vi "CCD_config.vi"() -> ()   [LabVIEW 2014]
uses:
  Public/Documents/SIToolkit/LabVIEW/Examples2014_6_0_2_9/Fast Examples/Open-Close Hardware/CamHandle.vi
  <vilib>/Utility/file.llb/Write To Spreadsheet File (I64).vi
  <vilib>/Utility/file.llb/Write To Spreadsheet File (DBL).vi
panel:
  in  "?":enum32{"CONFIGERATION", "OPERATION"}(tab)
  in  "Bypass Cooling":bool
  out "Camera Open":bool=TRUE
  in  "Write Tab Control":T1(tab)=enum."ROI"
  in  "Frames to collect (nframe)":u32=1 min=1 step=1
  in  "Exposure":dbl min=0.0 step=0.001 format="%.3f"
  in  "Timing Mode":u32(ring)=3 items=["Free Run/Timed"=1, "External Sync"=3, "Shift per Trigger"=13]
  in  "Trigger Edge":u32(ring)=1 items=["Positive Edge"=1, "Negative Edge"=2]
  in  "Collection Mode":u32(ring)=1 items=["Focus"=1, "N-Frame"=2, "Asynchronous"=3]
  in  "ReadOut Mode":u16(ring)=1 items=["Full Frame"=1, "Kinetics"=10]
  in  "Temperature":dbl=-75.0 format="%.2f"
  in  "Speed":i32=-2 min=-3 step=1
  in  "Gain":i32(ring)=1 items=["Don't Change "=-1, "Low"=1, "Medium"=2, "High"=3]
  in  "Offset":i32=-1 min=-1 step=1
  in  "Readout Port":i32(ring)=2 items=["Don't Change"=-1, "Low Noise"=1, "High capacity"=2]
  in  "Open":u32
  in  "Close":u32
  in  "Shutter State":u16(ring)=3 items=["Always Closed"=1, "Open Each Exposure"=2, "Open at Begining of Acquisition"=3, "Open While Waiting for Trigger"=4]
  in  "Final Section Height\n(Minimum Block Size)":u32=100
  in  "Final Section Count\n(Number of Minimum Blocks)":u32=10
  in  "Number of Clean/Clears cycles":u32
  in  "Clean cycle height (Number of \nStrips per Clean/Clear)":u32=100
  in  "Continous Cleans":bool
  in  "Skip Serial Register Clean":bool
  in  "Kinetics Window Height":u32
  in  "Active Y Size":u32=100
  in  "Post Y":u32=8
  in  "Pre Y":u32=8
  in  "Active X Size":u32=1340
  in  "Post X":u32
  in  "Pre X":u32
  in  "Vertical Timing Index":u32
  in  "Enable / Disable Custom Chip":bool
  in  "Logic Output":u16(ring)=3 items=["Not Scan / Not Reading"=1, "Shutter Open"=2, "Not Ready/Busy"=3, "Always Low"=4, "Always High"=8]
  in  "Invert":bool
  out "Y Size ROI":u32=100
  out "X Size ROI":u32=1340
  in  "Y Bin":u32=100 min=1 step=1
  in  "Y End":u32=100 min=1 step=1
  in  "Y Start":u32=1 min=1 step=1
  in  "X Bin":u32=1 min=1 step=1
  in  "X End":u32=1340 min=1 max=100000 step=1
  in  "X Start":u32=1 min=1 step=1
  in  "Camera Number":u32=1
  in  "Error Codes":string="Ready"
  out "Frame Rate Calc":dbl=1001.0010010010011
  out "Vertical Index":u32
  out "Custom Chip Enabled":bool
  out "Vertical Timing":dbl=3.2
  out "Readout Time":dbl=0.9989999999999999
  out "Temperature":dbl=-66.0
  out "Pixel Time\n(1/ADC Speed)":i32=500
  out "Bit Depth":i32=16
  out "ReadOut Port":i32=2
  out "ADC Offset":i32=-1
  out "ADC Gain":i32=1
  out "ADC Speed":i32=2000
  in  "error in (no error)":errorcluster
  out "error out":errorcluster
  out "Camera Handle":u32
  in  "INI Flag":bool=TRUE
  in  "Run":enum32{"RUN", "FOCUS", "FSRS", "SPECTROGRAPH"}(tab)
  in  "?":bool
  in  "Exposure Time (s)":dbl=0.004 min=0.0 step=0.001 format="%.3f"
  in  "?":bool
  in  "?":bool
  out "?":u16[](graph)
  in  "file path":path
  in  "File_name":string
  in  "# of spectrum per frame":i32
  in  "# of Frames":i32
  out "Gain":dbl
  in  "FLIP SPECTRA":bool
  in  "?":bool
  in  "?":bool
  in  "?":bool
  out "Spectra":dbl[](graph)
  in  "?":bool
  in  "Number of Images":u32=1 min=1 step=1
  out "DATA LOOP":dbl
  out "?":dbl[](graph)
  in  "?":bool
  in  "# of Sets":i32
  out "Current Set":u32=24
  in  "#Ground per set":u32=3
  in  "Timepoints":dbl[](array[numeric])=[200.0, 100.0, 300.0, 400.0, 500.0]
  in  "File Path":path
  in  "File Name":string
  in  "Ground State\nSubstract?":bool
  in  "?":bool
  out "Ready to Run":bool
  # "Timing"
  # "Seconds"
  # "Temperature"
  # "°C"
  # "ADC"
  # "-3 = SLOWEST speed\n-2 = FASTEST speed\n-1 = CURRENT speed (or do not wire)\nOtherwise enter speed in kHz"
  # "Shutter"
  # "Compensation Times"
  # "ms"
  # "Cleans / Clears"
  # "Custom Chip and Timing"
  # "Valid When Kinetics Timing Mode Active"
  # "Logic Output"
  # "Region Of Interest"
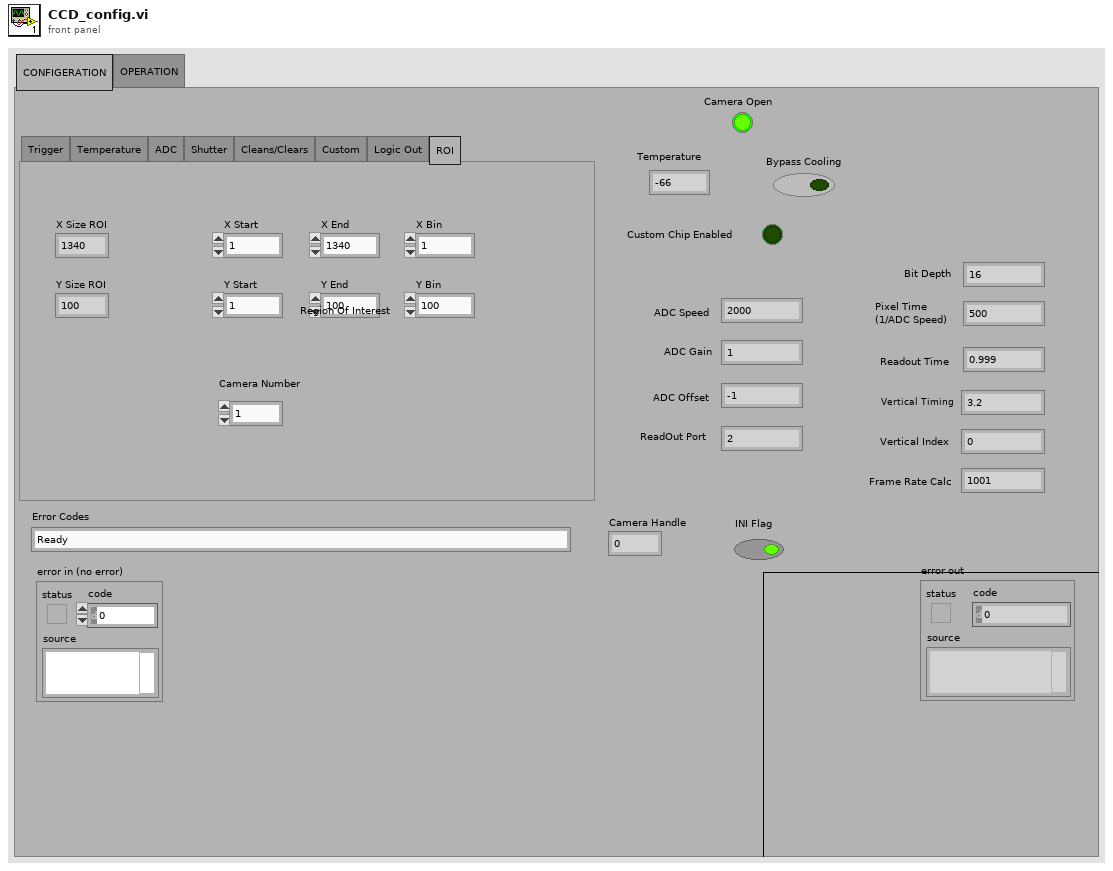
[diagram p1: front panel]
types:
  T1 = enum32{"Trigger", "Temperature", "ADC", "Shutter", "Cleans/Clears", "Custom", "Logic Out", "ROI"}
  T2 = enum8{"Enabled", "Disabled", "Disabled and Grayed Out"}
  T3 = cluster{"Camera Number":i32, "ROI Number":i32, "X Start":i32, "X End":i32, "X Bin":i32, "Y Start":i32, "Y End":i32, "Y Bin":i32}
  T4 = cluster{"Pre Y":u32, "Post Y":u32, "Active Y":u32, "Pre X":u32, "Post X":u32, "Active X":u32, "Custom Chip Enabled":bool, "Vertical Timing Index":u32}
  T5 = cluster{"Exposure":dbl, "Collection Mode":u32, "Timing Mode":u32, "Trigger Edge":u32, "Temperature":dbl}
  T6 = cluster{"ADC Speed":i32, "ADC Gain":i32, "ADC Offset":i32, "Readout Port":i32, "Num Cleans":u32, "Num Strips per Clean":u32, "Mini Block Size":u32, "Num Min Blocks":u32, "Continous Cleans":bool, "Skip Serial Reg Clean":bool}
  T7 = cluster{"Shutter State":u16, "Open Comp Time ":u32, "Close Comp Time":u32, "Logic Out Setting":u32, "Logic Out Invert":bool}
  T8 = cluster{"acquire focus mode":u32, "Exposure Time (s)":dbl, i32, "Software accumulation":u32}
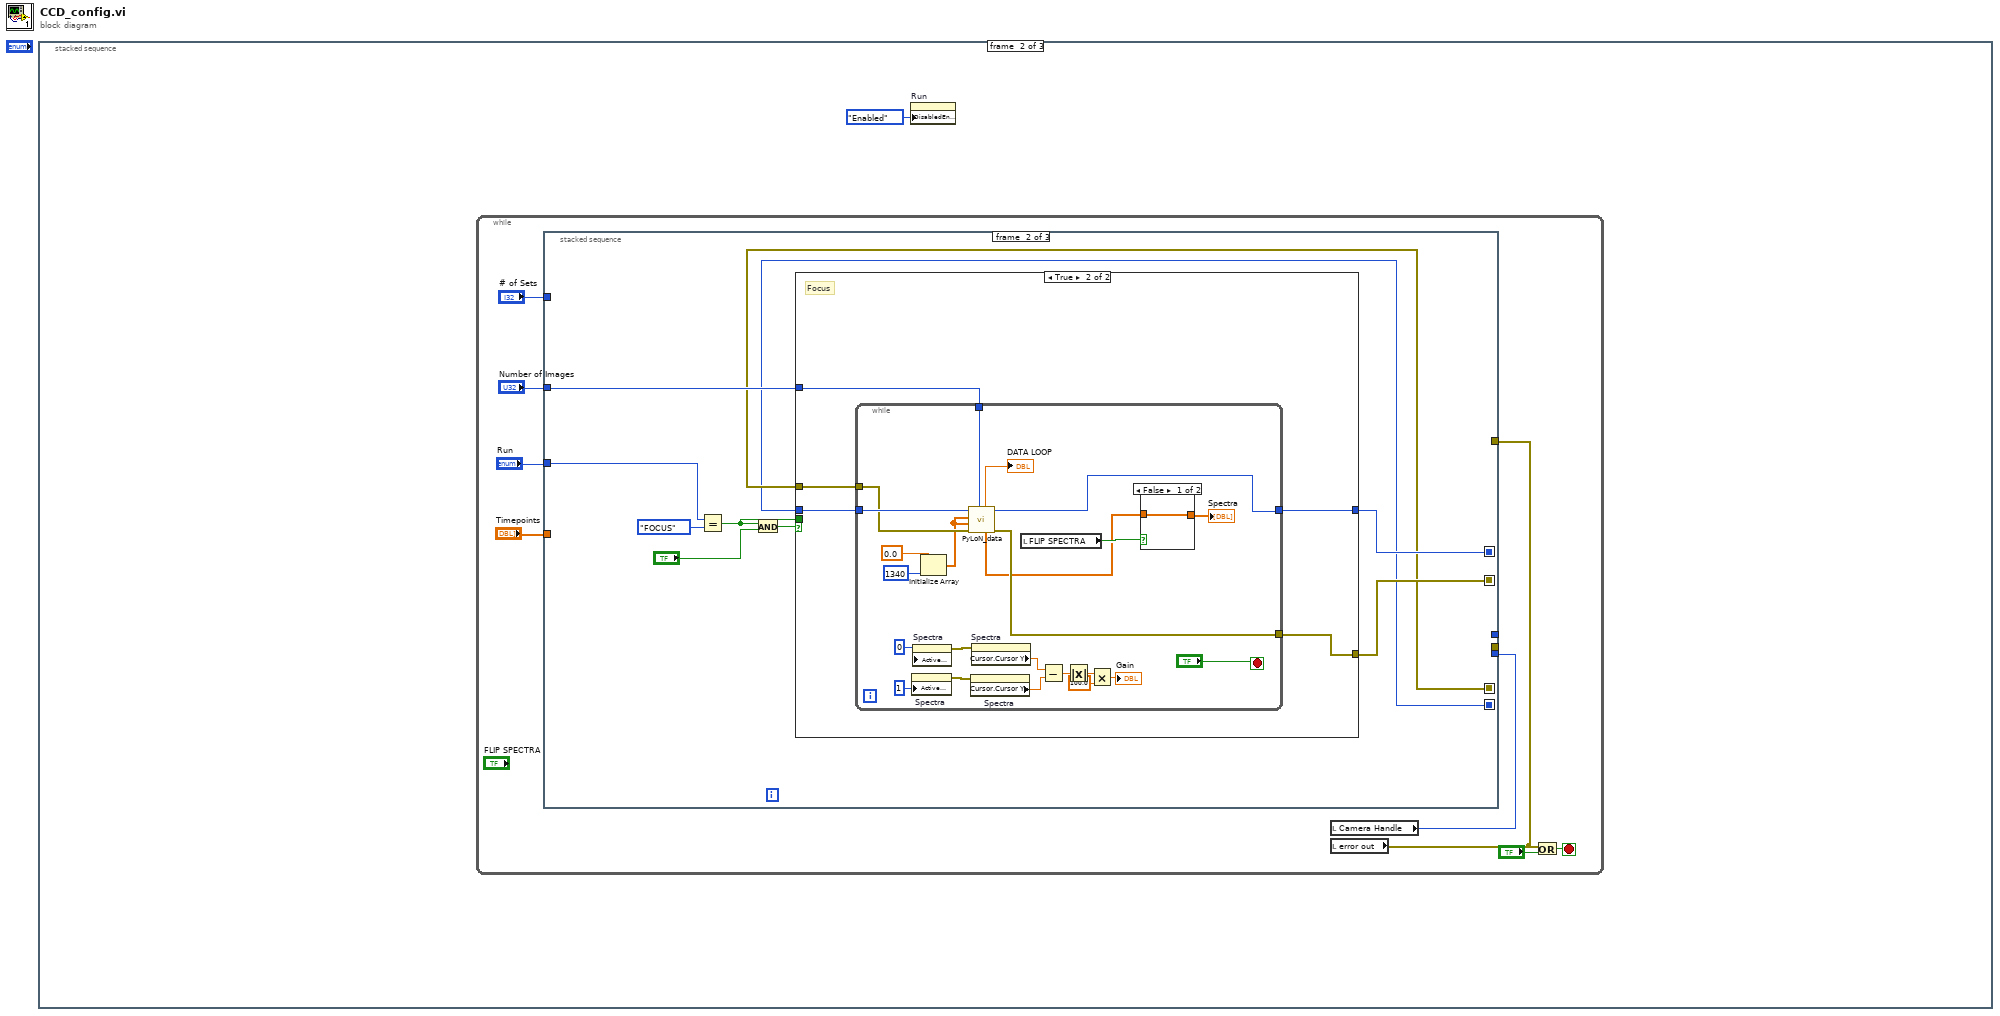
[diagram p0: block diagram]
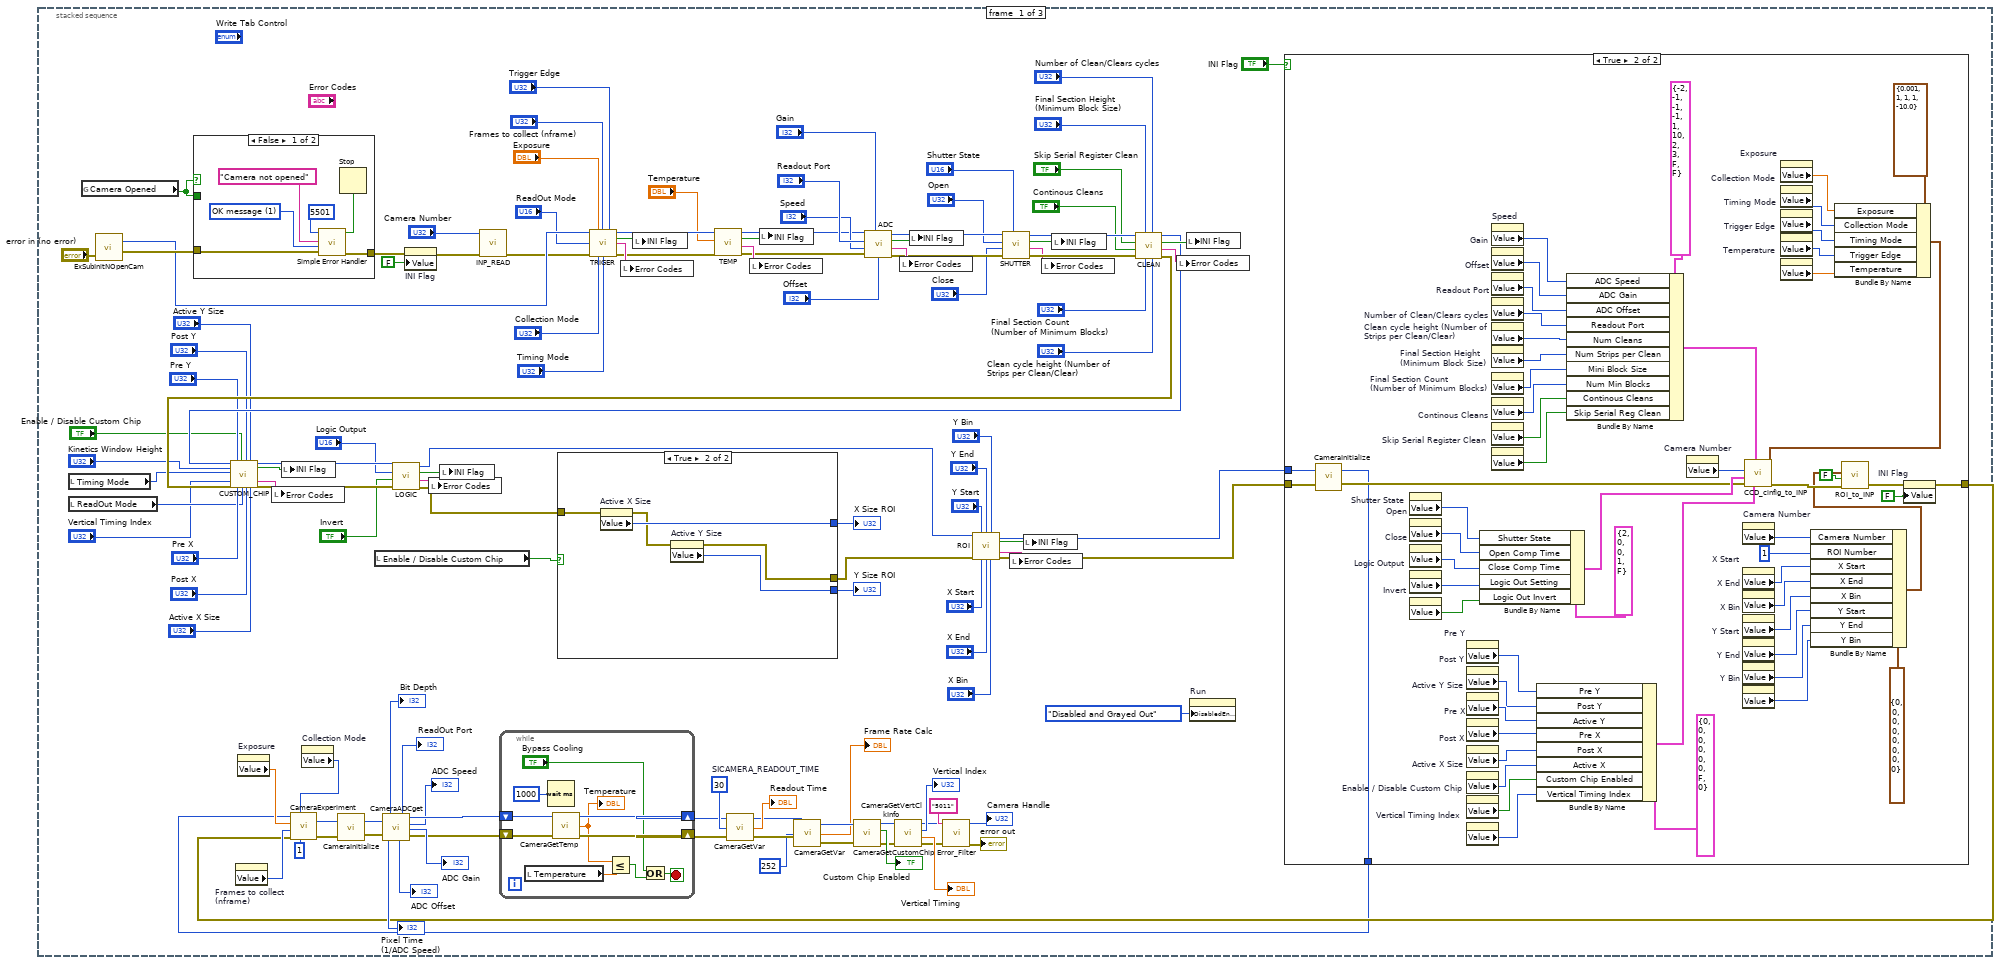
[diagram p2: hidden frame]
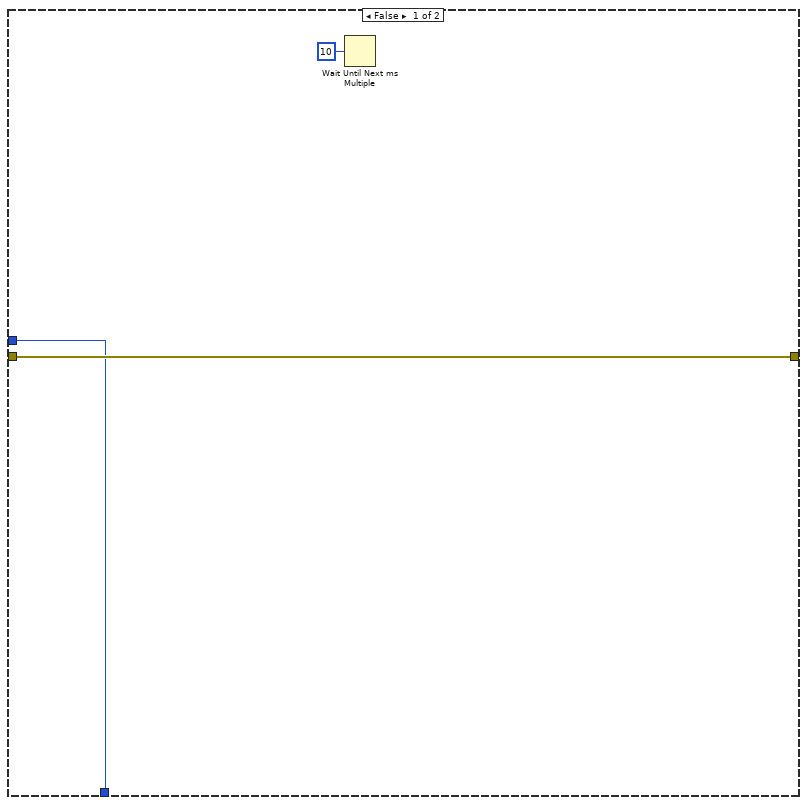
[diagram p3: hidden frame]
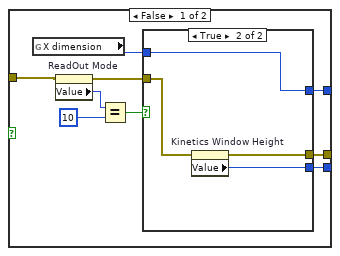
[diagram p4: hidden frame]
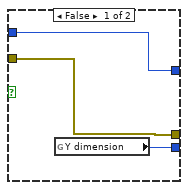
[diagram p5: hidden frame]
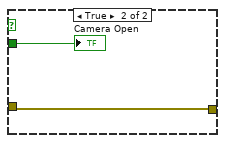
[diagram p6: hidden frame]
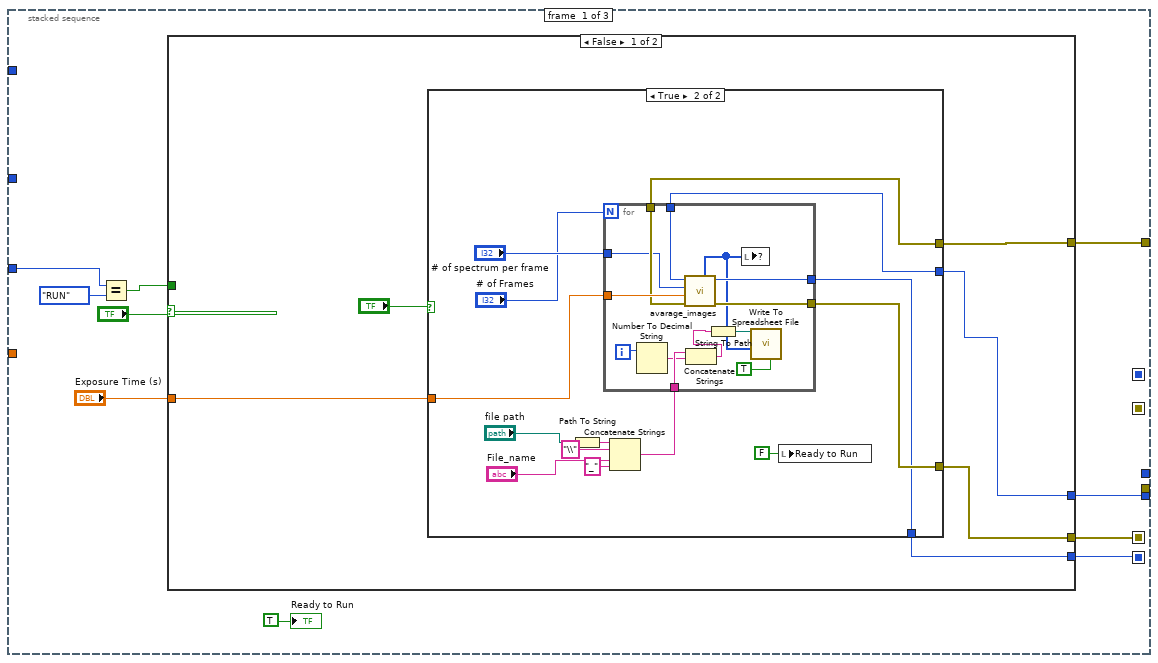
[diagram p7: hidden frame]
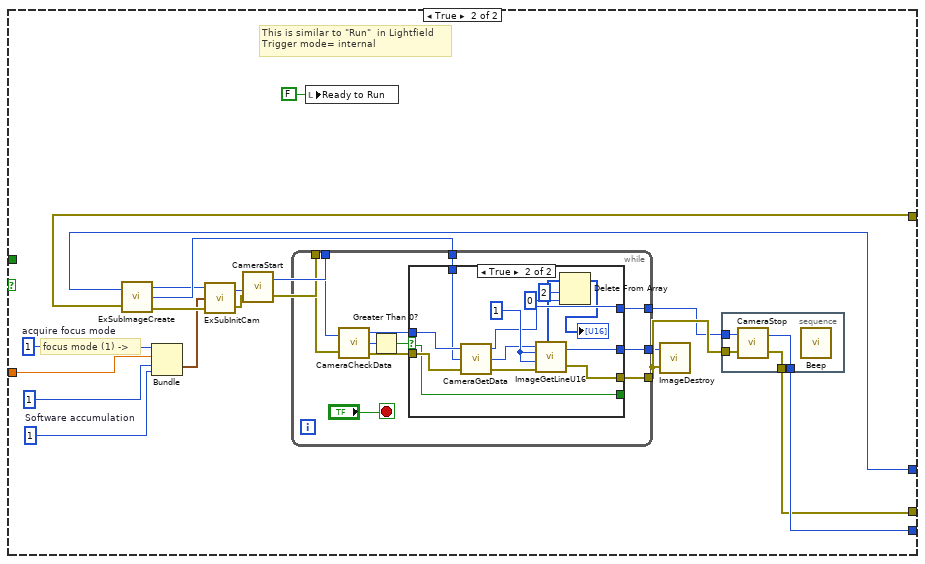
[diagram p9: hidden frame]
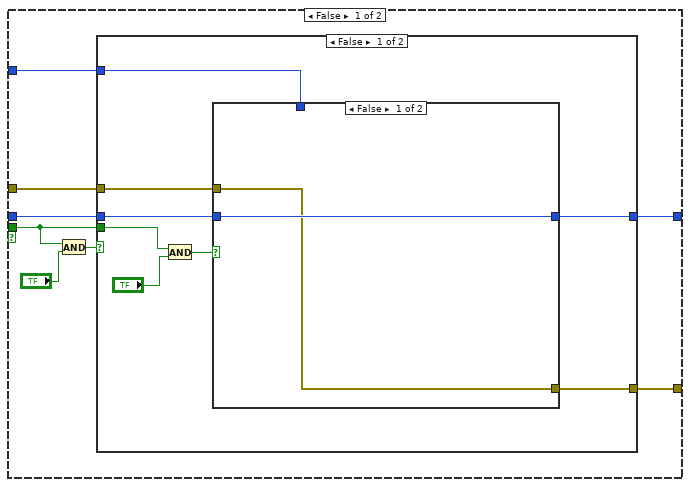
[diagram p11: hidden frame]
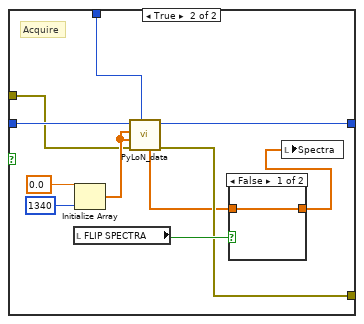
[diagram p12: hidden frame]
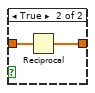
[diagram p13: hidden frame]
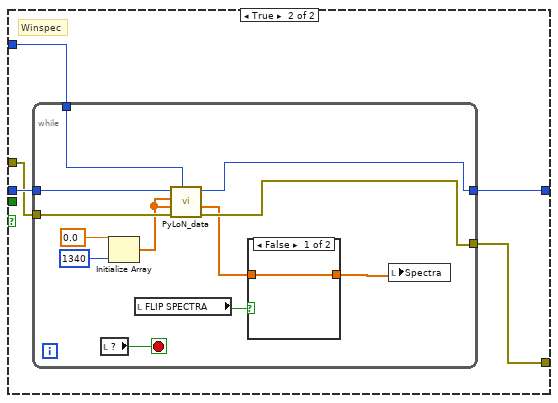
[diagram p14: hidden frame]
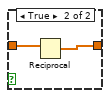
[diagram p15: hidden frame]
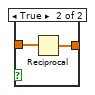
[diagram p16: hidden frame]
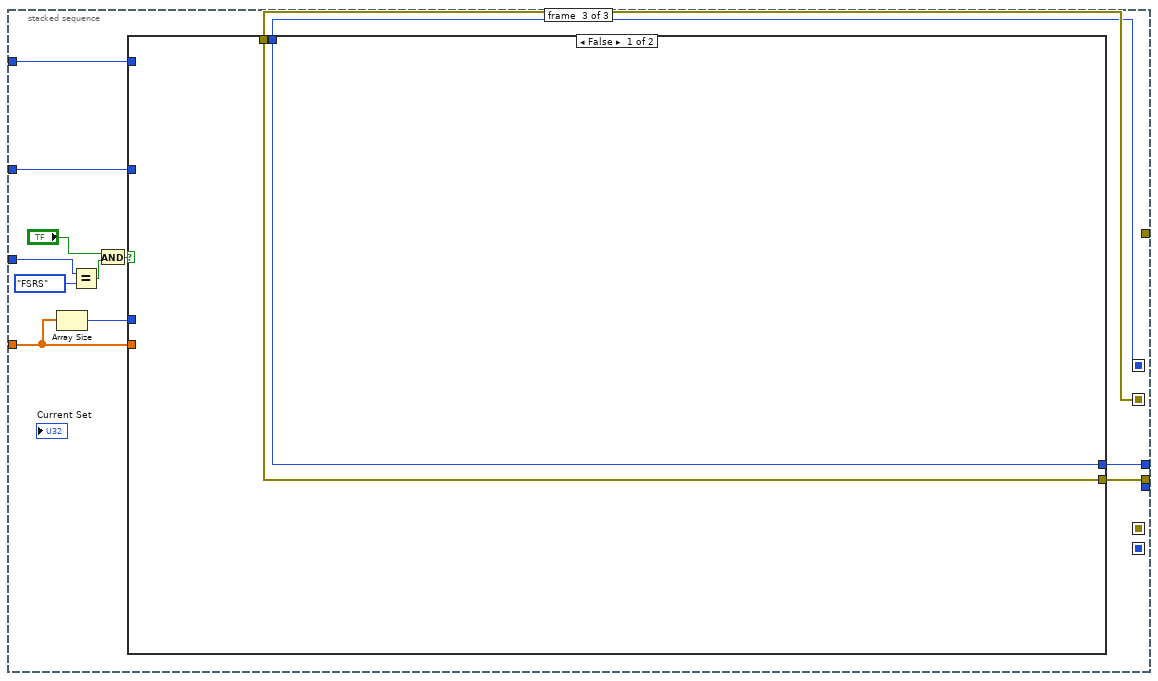
[diagram p17: hidden frame]
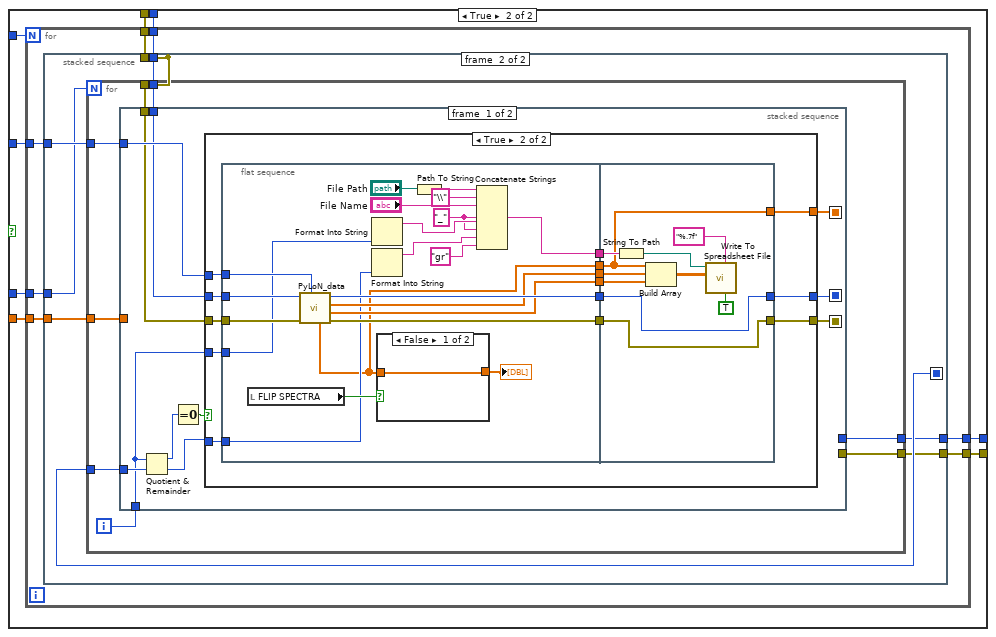
[diagram p18: hidden frame]
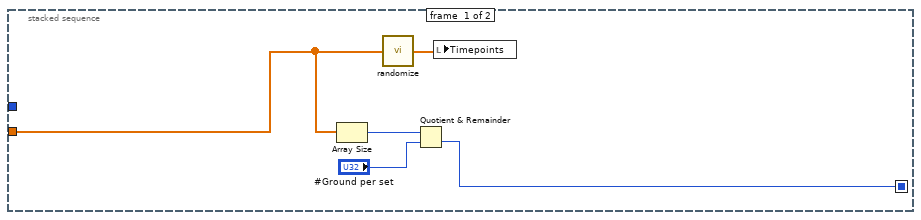
[diagram p19: hidden frame]
diagram:
  n1 = stacked-sequence {
    frame #0 {
      w33 = 30  # SICAMERA_READOUT_TIME
      n2 = local read "Timing Mode"() -> (w64:u32)
      n3 = local read "ReadOut Mode"() -> (w65:u16)
      n4 = global read "CamHandle.vi" "Camera Opened"() -> (w121:bool)
      n5 = call "ExSubInitNOpenCam.vi"("error in (no error)"="error in (no error)") -> ("Camera Handle"=w118:u32, "error out"=w119:errorcluster)
      n6 = case shown="False" w121 {
        tunnel: [w219 w221] -> w123
        tunnel: w119 -> [w215 w221]
        tunnel: w121 -> [_ w220]
        frame False {
          w214 = u16 1 items=["no dialog", "OK message", "continue or stop message"] ("type of dialog (OK msg:1)")
          n7 = call <vilib>:"Simple Error Handler.vi"("error code (no error:0)"=5501, "error source (\" \")"="Camera not opened", "type of dialog (OK msg:1)"=w214, "error in (no error)"=w215) -> ("error?"=w217:bool, "error out"=w219:errorcluster)  [unwired: 1 in, 3 out]
          n8 = Stop(stop? (T)=w217) -> ()
        }
        frame True {
          "Camera Open" <- w220
        }
      }
      n9 = property on="Frames to collect (nframe)" class="DigNum (strict)"() -> ("Value"=w11:u32)  [unwired: 2 in, 2 out]
      n10 = property on="Exposure" class="DigNum (strict)"() -> ("Value"=w14:dbl)  [unwired: 2 in, 2 out]
      n11 = property on="Collection Mode" class="Ring (strict)"() -> ("Value"=w9:u32)  [unwired: 2 in, 2 out]
      n12 = local read "Enable / Disable Custom Chip"() -> (w55:bool)
      n13 = property on="INI Flag" class="Bool (strict)"(error in=w123, "Value"=FALSE) -> (error out=w103:errorcluster)  [unwired: 1 in, 1 out]
      n14 = call "INP_READ.vi"("error in (no error)"=w103, "Camera Number"="Camera Number") -> ("error out"=w102:errorcluster)  [unwired: 4 in, 5 out]
      n15 = call "TRIGER.vi"("Camera Handle"=w118, "Exposure (sec)"="Exposure", "Number of frams"="Frames to collect (nframe)", "Trigger Edge"="Trigger Edge", "ReadOut Mode"="ReadOut Mode", "error out"=w102, "Acquire / Focus Flag"="Collection Mode", "Timing Mode"="Timing Mode") -> ("Camera Handle"=w109:u32, "INI Flag"=w111:bool, "String"=w110:string, "error out"=w108:errorcluster)  [unwired: 4 in]
      n16 = local write "Error Codes"(w110) -> ()
      n17 = local write "INI Flag"(w111) -> ()
      n18 = call "TEMP.vi"("error in (no error)"=w108, "Temperature"="Temperature", "Camera Handle"=w109) -> ("error out"=w99:errorcluster, "String"=w106:string, "INI Flag"=w105:bool, "Camera Handle"=w94:u32)  [unwired: 5 in]
      n19 = local write "Error Codes"(w106) -> ()
      n20 = local write "INI Flag"(w105) -> ()
      n21 = call "ADC.vi"("ADC offset"="Offset", "ADC Gain"="Gain", "error in (no error)"=w99, "ADC Speed"="Speed", "Read Out port"="Readout Port", "Camera Handle"=w94) -> ("error out"=w92:errorcluster, "string"=w95:string, "INI Flag"=w96:bool, "Camera Handle"=w93:u32)  [unwired: 2 in]
      n22 = local write "Error Codes"(w95) -> ()
      n23 = local write "INI Flag"(w96) -> ()
      n24 = call "SHUTTER.vi"("Shutter State"="Shutter State", "error out"=w92, "Shutter Comp Time: Pre Open"="Close", "Shutter Comp Time: Post Open"="Open", "Camera Handle"=w93) -> ("error out"=w87:errorcluster, "String"=w86:string, "INI Flag"=w85:bool, "Camera Handle"=w88:u32)  [unwired: 3 in]
      n25 = local write "Error Codes"(w86) -> ()
      n26 = local write "INI Flag"(w85) -> ()
      n27 = call "CLEAN.vi"("Number of Strips Per Clear"="Clean cycle height (Number of \nStrips per Clean/Clear)", "Number of Clears"="Number of Clean/Clears cycles", "Number of Minimum blocks"="Final Section Count\n(Number of Minimum Blocks)", "Minimum Block Size"="Final Section Height\n(Minimum Block Size)", "error out"=w87, "Continous Clean"="Continous Cleans", "Skip Serial Reg Clean"="Skip Serial Register Clean", "Camera Handle"=w88) -> ("error out 2"=w75:errorcluster, "String"=w78:string, "INI Flag"=w77:bool, "CameraHandle"=w76:u32)
      n28 = call "CUSTOM_CHIP.vi"("Camera Handle"=w76, "Window Size"="Kinetics Window Height", "TriggerMode"=w64, "Vertical Clock"="Vertical Timing Index", "error out"=w75, "Pre Y"="Pre Y", "Pre X"="Pre X", "Enable / Disable Custom Chip"="Enable / Disable Custom Chip", "ReadOut Mode"=w65, "Post Y"="Post Y", "Post X"="Post X", "Parallel (Y) Size"="Active Y Size", "Serial (X) Size"="Active X Size") -> ("Camera Handle"=w61:u32, "INI Flag"=w67:bool, "String"=w66:string, "error out"=w60:errorcluster)  [unwired: 3 in]
      n29 = local write "Error Codes"(w66) -> ()
      n30 = local write "INI Flag"(w67) -> ()
      n31 = call "LOGIC.vi"("error out"=w60, "Invert"="Invert", "Logic Output"="Logic Output", "Camera Handle"=w61) -> ("error out 2"=w54:errorcluster, "String"=w56:string, "INI Flag"=w57:bool, "Camera Handle"=w53:u32)  [unwired: 4 in]
      n32 = local write "Error Codes"(w56) -> ()
      n33 = local write "INI Flag"(w57) -> ()
      n34 = case shown="True" w55 {
        tunnel: [w197 w213] -> w44
        tunnel: [w196 w212] -> w45
        tunnel: w54 -> [w194 w210]
        tunnel: [w195 w209] -> w52
        frame False {
          n35 = global read "CamHandle.vi" "X dimension"() -> (w198:u32)
          n36 = property on="ReadOut Mode" class="Ring (strict)"(error in=w194) -> (error out=w193:errorcluster, "Value"=w199:u16)  [unwired: 1 in, 1 out]
          n37 = Equal?(x=w199, y=10) -> (x = y?=w200:bool)
          n38 = case shown="True" w200 {
            tunnel: w198 -> [w204 w208]
            tunnel: [w204 w208] -> w197
            tunnel: [w203 w207] -> w196
            tunnel: [w202 w206] -> w195
            tunnel: w193 -> [w202 w205]
            frame False {
              n39 = global read "CamHandle.vi" "Y dimension"() -> (w203:u32)
            }
            frame True {
              n40 = property on="Kinetics Window Height" class="DigNum (strict)"(error in=w205) -> (error out=w206:errorcluster, "Value"=w207:u32)  [unwired: 1 in, 1 out]
            }
          }
        }
        frame True {
          n41 = property on="Active X Size" class="DigNum (strict)"(error in=w210) -> (error out=w211:errorcluster, "Value"=w213:u32)  [unwired: 1 in, 1 out]
          n42 = property on="Active Y Size" class="DigNum (strict)"(error in=w211) -> (error out=w209:errorcluster, "Value"=w212:u32)  [unwired: 1 in, 1 out]
        }
      }
      "X Size ROI" <- w44
      "Y Size ROI" <- w45
      n43 = call "ROI.vi"("Camera Handle"=w53, "Y Start"="Y Start", "Y End"="Y End", "Y Bin"="Y Bin", "error in"=w52, "X Start"="X Start", "X End"="X End", "X Bin"="X Bin") -> ("Camera Handle"=w6:u32, "INI Flag"=w42:bool, "String"=w43:string, "error out"=w5:errorcluster)  [unwired: 4 in]
      n44 = local write "Error Codes"(w43) -> ()
      n45 = local write "INI Flag"(w42) -> ()
      n46 = local write "Error Codes"(w78) -> ()
      n47 = local write "INI Flag"(w77) -> ()
      n48 = property on="Run" class="TabCtl (strict)"("DisabledEnum"=T2."Disabled and Grayed Out" ("Disabled")) -> ()  [unwired: 2 in, 2 out]
      n49 = case shown="True" "INI Flag" {
        tunnel: w5 -> [w136 w164]
        tunnel: [w136 w162] -> w7
        tunnel: w6 -> [w134 w138]
        tunnel: [w134 w137] -> w4
        frame False {
          n50 = Wait Until Next ms Multiple(millisecond multiple=u32 10) -> ()  [unwired: 1 out]
        }
        frame True {
          n51 = call <userlib>:"CameraInitialize.vi"("error in"=w164, "Camera Handle"=w138) -> ("error out"=w165:errorcluster, "Camera Handle"=w137:u32)
          n52 = property on="Shutter State" class="Ring (strict)"() -> ("Value"=w186:u16)  [unwired: 2 in, 2 out]
          n53 = property on="Open" class="DigNum (strict)"() -> ("Value"=w187:u32)  [unwired: 2 in, 2 out]
          n54 = property on="Close" class="DigNum (strict)"() -> ("Value"=w188:u32)  [unwired: 2 in, 2 out]
          n55 = property on="Logic Output" class="Ring (strict)"() -> ("Value"=w189:u16)  [unwired: 2 in, 2 out]
          n56 = property on="Invert" class="Bool (strict)"() -> ("Value"=w190:bool)  [unwired: 2 in, 2 out]
          n57 = property on="Pre Y" class="DigNum (strict)"() -> ("Value"=w159:u32)  [unwired: 2 in, 2 out]
          n58 = property on="Post Y" class="DigNum (strict)"() -> ("Value"=w151:u32)  [unwired: 2 in, 2 out]
          n59 = property on="Active Y Size" class="DigNum (strict)"() -> ("Value"=w154:u32)  [unwired: 2 in, 2 out]
          n60 = property on="Pre X" class="DigNum (strict)"() -> ("Value"=w158:u32)  [unwired: 2 in, 2 out]
          n61 = property on="Post X" class="DigNum (strict)"() -> ("Value"=w152:u32)  [unwired: 2 in, 2 out]
          n62 = property on="Active X Size" class="DigNum (strict)"() -> ("Value"=w157:u32)  [unwired: 2 in, 2 out]
          n63 = property on="Enable / Disable Custom Chip" class="Bool (strict)"() -> ("Value"=w156:bool)  [unwired: 2 in, 2 out]
          n64 = property on="Vertical Timing Index" class="DigNum (strict)"() -> ("Value"=w155:u32)  [unwired: 2 in, 2 out]
          n65 = Bundle By Name(cluster=T7 {"Shutter State"=2, "Open Comp Time "=0, "Close Comp Time"=0, "Logic Out Setting"=1, "Logic Out Invert"=FALSE} ("Shutter and Logic Out"), "Shutter State"=w186, "Open Comp Time"=w187, "Close Comp Time"=w188, "Logic Out Setting"=w189, "Logic Out Invert"=w190) -> (w191:T7)
          n66 = property on="Speed" class="DigNum (strict)"() -> ("Value"=w183:i32)  [unwired: 2 in, 2 out]
          n67 = property on="Gain" class="Ring (strict)"() -> ("Value"=w182:i32)  [unwired: 2 in, 2 out]
          n68 = property on="Offset" class="DigNum (strict)"() -> ("Value"=w180:i32)  [unwired: 2 in, 2 out]
          n69 = property on="Readout Port" class="Ring (strict)"() -> ("Value"=w178:i32)  [unwired: 2 in, 2 out]
          n70 = property on="Number of Clean/Clears cycles" class="DigNum (strict)"() -> ("Value"=w177:u32)  [unwired: 2 in, 2 out]
          n71 = property on="Clean cycle height (Number of \nStrips per Clean/Clear)" class="DigNum (strict)"() -> ("Value"=w176:u32)  [unwired: 2 in, 2 out]
          n72 = property on="Final Section Height\n(Minimum Block Size)" class="DigNum (strict)"() -> ("Value"=w174:u32)  [unwired: 2 in, 2 out]
          n73 = property on="Final Section Count\n(Number of Minimum Blocks)" class="DigNum (strict)"() -> ("Value"=w175:u32)  [unwired: 2 in, 2 out]
          n74 = property on="Continous Cleans" class="Bool (strict)"() -> ("Value"=w179:bool)  [unwired: 2 in, 2 out]
          n75 = property on="Skip Serial Register Clean" class="Bool (strict)"() -> ("Value"=w181:bool)  [unwired: 2 in, 2 out]
          n76 = Bundle By Name(cluster=T4 {"Pre Y"=0, "Post Y"=0, "Active Y"=0, "Pre X"=0, "Post X"=0, "Active X"=0, "Custom Chip Enabled"=FALSE, "Vertical Timing Index"=0} ("Custom Chip"), "Pre Y"=w159, "Post Y"=w151, "Active Y"=w154, "Pre X"=w158, "Post X"=w152, "Active X"=w157, "Custom Chip Enabled"=w156, "Vertical Timing Index"=w155) -> (w153:T4)
          n77 = Bundle By Name(cluster=T6 {"ADC Speed"=-2, "ADC Gain"=-1, "ADC Offset"=-1, "Readout Port"=-1, "Num Cleans"=1, "Num Strips per Clean"=10, "Mini Block Size"=2, "Num Min Blocks"=3, "Continous Cleans"=FALSE, "Skip Serial Reg Clean"=FALSE} ("ADC and Cleans"), "ADC Speed"=w183, "ADC Gain"=w182, "ADC Offset"=w180, "Readout Port"=w178, "Num Cleans"=w177, "Num Strips per Clean"=w176, "Mini Block Size"=w174, "Num Min Blocks"=w175, "Continous Cleans"=w179, "Skip Serial Reg Clean"=w181) -> (w184:T6)
          n78 = property on="Camera Number" class="DigNum (strict)"() -> ("Value"=w166:u32)  [unwired: 2 in, 2 out]
          n79 = property on="Camera Number" class="DigNum (strict)"() -> ("Value"=w148:u32)  [unwired: 2 in, 2 out]
          n80 = property on="X Start" class="DigNum (strict)"() -> ("Value"=w146:u32)  [unwired: 2 in, 2 out]
          n81 = property on="X End" class="DigNum (strict)"() -> ("Value"=w145:u32)  [unwired: 2 in, 2 out]
          n82 = property on="X Bin" class="DigNum (strict)"() -> ("Value"=w144:u32)  [unwired: 2 in, 2 out]
          n83 = property on="Y Start" class="DigNum (strict)"() -> ("Value"=w143:u32)  [unwired: 2 in, 2 out]
          n84 = property on="Y End" class="DigNum (strict)"() -> ("Value"=w142:u32)  [unwired: 2 in, 2 out]
          n85 = property on="Y Bin" class="DigNum (strict)"() -> ("Value"=w141:u32)  [unwired: 2 in, 2 out]
          n86 = property on="Exposure" class="DigNum (strict)"() -> ("Value"=w167:dbl)  [unwired: 2 in, 2 out]
          n87 = property on="Collection Mode" class="Ring (strict)"() -> ("Value"=w168:u32)  [unwired: 2 in, 2 out]
          n88 = property on="Timing Mode" class="Ring (strict)"() -> ("Value"=w169:u32)  [unwired: 2 in, 2 out]
          n89 = property on="Trigger Edge" class="Ring (strict)"() -> ("Value"=w170:u32)  [unwired: 2 in, 2 out]
          n90 = property on="Temperature" class="DigNum (strict)"() -> ("Value"=w171:dbl)  [unwired: 2 in, 2 out]
          n91 = Bundle By Name(cluster=T3 {"Camera Number"=0, "ROI Number"=0, "X Start"=0, "X End"=0, "X Bin"=0, "Y Start"=0, "Y End"=0, "Y Bin"=0} ("ROI Values"), "Camera Number"=w148, "ROI Number"=1, "X Start"=w146, "X End"=w145, "X Bin"=w144, "Y Start"=w143, "Y End"=w142, "Y Bin"=w141) -> (w140:T3)
          n92 = Bundle By Name(cluster=T5 {"Exposure"=0.001, "Collection Mode"=1, "Timing Mode"=1, "Trigger Edge"=1, "Temperature"=-10.0} ("Timing and Temperature"), "Exposure"=w167, "Collection Mode"=w168, "Timing Mode"=w169, "Trigger Edge"=w170, "Temperature"=w171) -> (w172:T5)
          n93 = call "CCD_cinfig_to_INP.vi"("Timing and Temperature"=w172, "Custom Chip"=w153, "ADC and Cleans"=w184, "error in (no error)"=w165, "Shutter and Logic Out"=w191, "Camera Number"=w166) -> ("error out"=w163:errorcluster)  [unwired: 5 in]
          n94 = call "ROI_to_INP.vi"("error in (no error)"=w163, "Show Message"=FALSE, "ROI Values"=w140) -> ("error out"=w150:errorcluster)  [unwired: 8 in]
          n95 = property on="INI Flag" class="Bool (strict)"(error in=w150, "Value"=FALSE) -> (error out=w162:errorcluster)  [unwired: 1 in, 1 out]
        }
      }
      n96 = call <userlib>:"CameraExperiment.vi"("Number of Accumulations"=1, "Acquire / Focus Flag"=w9, "error in"=w7, "Number of Images"=w11, "Exposure (sec)"=w14, "Camera Handle"=w4) -> ("error out"=w16:errorcluster, "Camera Handle"=w15:u32)
      n97 = call <userlib>:"CameraInitialize.vi"("error in"=w16, "Camera Handle"=w15) -> ("error out"=w18:errorcluster, "Camera Handle"=w17:u32)
      n98 = call <userlib>:"CameraADCget.vi"("Camera handle"=w17, "error in (no error)"=w18) -> ("Bit Depth"=→"Bit Depth":i32, "Pixel Time"=→"Pixel Time\n(1/ADC Speed)":i32, "Readout Port"=→"ReadOut Port":i32, "ADC Offset"=→"ADC Offset":i32, "Camera handle"=w34:u32, "ADC Speed"=→"ADC Speed":i32, "ADC Gain"=→"ADC Gain":i32, "error out"=w35:errorcluster)
      n99 = while {
        shift-right: [w131] -> w32
        shift-left: w35 -> [w133]
        shift-right: [w130] -> w31
        shift-left: w34 -> [w132]
        stop <- w126 stop-if-true
        n100 = local read "Temperature"() -> (w128:dbl)
        n101 = Wait (ms)(milliseconds to wait=u32 1000) -> ()  [unwired: 1 out]
        n102 = call <userlib>:"CameraGetTemp.vi"("Camera Handle"=w132, "error in (no error)"=w133) -> ("Camera Handle"=w130:u32, "Temperature"=w129:dbl, "error out"=w131:errorcluster)
        "Temperature" <- w129
        n103 = Less Or Equal?(x=w129, y=w128) -> (x <= y?=w124:bool)
        n104 = Or(x="Bypass Cooling", y=w124) -> (x .or. y?=w126:bool)
      }
      n105 = call <userlib>:"CameraGetVar.vi"("error in"=w32, "Parameter ID"=w33, "Camera Handle"=w31) -> ("error out"=w24:errorcluster, "Value"=→"Readout Time":dbl, "Camera Handle"=w22:u32)
      n106 = call <userlib>:"CameraGetVar.vi"("error in"=w24, "Parameter ID"=252, "Camera Handle"=w22) -> ("error out"=w23:errorcluster, "Value"=→"Frame Rate Calc":dbl, "Camera Handle"=w21:u32)
      n107 = call <userlib>:"CameraGetCustomChip.vi"("Camera Handle"=w21, "error in (no error)"=w23) -> ("Camera Handle"=w28:u32, "Custum chip Enable/Disable status"=→"Custom Chip Enabled":bool, "error out"=w27:errorcluster)  [unwired: 1 out]
      n108 = call <userlib>:"CameraGetVertClkInfo.vi"("Camera Handle"=w28, "error in (no error)"=w27) -> ("Camera Handle"=→"Camera Handle":u32, "VertClk index"=→"Vertical Index":u32, "Real Clock Value"=→"Vertical Timing":dbl, "error out"=w13:errorcluster)  [unwired: 2 out]
      n109 = call "Error_Filter.vi"("error in (no error)"=w13, "Error Numbers To Filter"="5011") -> ("error out"=→"error out":errorcluster)  [unwired: 9 in]
    }
    frame #1 {
      n110 = while {
        stop <- w226 stop-if-true
        n111 = local read "Camera Handle"() -> (w223:u32)
        n112 = local read "error out"() -> (w224:errorcluster)
        n113 = stacked-sequence {
          seq-local: [_ w333 _] -> [_ _ w428]
          seq-local: [_ w332 _] -> [_ _ w430]
          seq-local: [w236 _ _] -> [_ w330 _]
          seq-local: [w237 _ _] -> [_ w331 _]
          tunnel: w223 -> [w234 _ _]
          tunnel: w224 -> [w240 _ _]
          tunnel: "Run" -> [w238 w338 w434]
          tunnel: "Number of Images" -> [_ w336 w431]
          tunnel: "Timepoints" -> [_ _ w424]
          tunnel: [_ _ w427] -> _
          tunnel: [_ _ w426] -> _
          tunnel: "# of Sets" -> [_ _ w425]
          frame #0 {
            n114 = Equal?(x=w238, y=enum32{"RUN", "FOCUS", "FSRS", "SPECTROGRAPH"}."RUN") -> (x = y?=w235:bool)
            n115 = case shown="False" "?" {
              tunnel: w240 -> [w246 w278]
              tunnel: [w243 w281] -> w236
              tunnel: [w245 w280] -> w237
              tunnel: w235 -> [_ _]
              tunnel: w234 -> [w244 w279]
              tunnel: "Exposure Time (s)" -> [w242 w276]
              frame False {
                n116 = case shown="True" "?" {
                  tunnel: w246 -> [w248 w260]
                  tunnel: [w248 w259] -> w245
                  tunnel: w244 -> [w247 w261]
                  tunnel: [w247 w258] -> w243
                  tunnel: w242 -> [_ w262]
                  frame False {
                  }
                  frame True {
                    n117 = Path To String(path="file path") -> (string=w254:string)
                    n118 = Concatenate Strings(w254, "\\" ("string"), "File_name", "_" ("string")) -> (w249:string)
                    n119 = for {
                      N: "# of Frames" -> [_]
                      tunnel: w262 -> [w275]
                      tunnel: w261 -> [w274]
                      tunnel: w260 -> [w273]
                      tunnel: [w272] -> w259
                      tunnel: [w271] -> w258
                      tunnel: "# of spectrum per frame" -> [w270]
                      tunnel: w249 -> [w266]
                      i -> [w263]
                      n120 = Number To Decimal String(number=w263) -> (decimal integer string=w265:string)  [unwired: 1 in]
                      n121 = call "avarage_images.vi"("error in (no error)"=w273, "Exposure Time (s)"=w275, "Number of Images"=w270, "Camera Handle"=w274) -> ("error out"=w272:errorcluster, "Camera Handle"=w271:u32, "Waveform Graph"=w269:i32[])  [unwired: 3 in, 2 out]
                      n122 = Concatenate Strings(w266, w265) -> (w264:string)
                      n123 = String To Path(string=w264) -> (path=w267:path)
                      n124 = local write item#16(w269) -> ()
                      n125 = call-poly <vilib>:"Write To Spreadsheet File.vi"("transpose? (no:F)"=TRUE, "1D data"=w269, "file path (dialog if empty)"=w267) -> ()  [unwired: 5 in, 1 out]
                    }
                    n126 = local write "Ready to Run"(FALSE ("PyLoN Ready")) -> ()
                  }
                }
              }
              frame True {
                w283 = u32 1  # acquire focus mode
                w284 = u32 1  # Software accumulation
                # "focus mode (1) ->"
                # "This is similar to \"Run\"  in Lightfield\nTrigger mode= internal"
                n127 = call "ExSubImageCreate.vi"("Camera Handle"=w279, "error in (no error)"=w278) -> ("Camera Handle"=w285:u32, "Data Handle"=w291:u32, "error out"=w286:errorcluster)
                n128 = Bundle("acquire focus mode"=w283, "Exposure Time (s)"=w276, 1, "Software accumulation"=w284) -> (w282:T8)  [unwired: 1 in]
                n129 = call "ExSubInitCam.vi"("error in (no error)"=w286, "Camera Information"=w282, "Camera Handle"=w285) -> ("error out"=w287:errorcluster, "Camera Handle"=w288:u32)
                n130 = call <userlib>:"CameraStart.vi"("error in"=w287, "Camera Handle"=w288) -> ("error out"=w289:errorcluster, "Camera Handle"=w290:u32)
                n131 = while {
                  tunnel: [w306] -> w292
                  tunnel: [w305] -> w294
                  tunnel: [w304] -> w293
                  tunnel: w289 -> [w303]
                  tunnel: w290 -> [w302]
                  tunnel: w291 -> [w301]
                  stop <- "?" stop-if-true
                  n132 = call <userlib>:"CameraCheckData.vi"("Camera Handle"=w302, "error in"=w303) -> ("Camera Handle"=w308:u32, "Number Of Frames Available"=w310:i32, "error out"=w307:errorcluster)
                  n133 = Greater Than 0?(x=w310) -> (x > 0?=w309:bool)
                  n134 = case shown="True" w309 {
                    selector: w309 -> [w313 w326]
                    tunnel: w308 -> [w311 w328]
                    tunnel: w307 -> [w314 w327]
                    tunnel: [w313 w326] -> _
                    tunnel: [w314 w325] -> w305
                    tunnel: w301 -> [w312 w319]
                    tunnel: [w312 w323] -> w306
                    tunnel: [w311 w322] -> w304
                    frame False {
                    }
                    frame True {
                      w324 = 1
                      n135 = call <userlib>:"CameraGetData.vi"("error in"=w327, "Image/Data Handle"=w319, "Camera Handle"=w328) -> ("error out"=w321:errorcluster, "Image/Data Handle"=w320:u32, "Camera Handle"=w322:u32)
                      n136 = call <userlib>:"ImageGetLineU16.vi"("Data Handle"=w320, "Y Position"=w324, "Z Position"=w324, "error in"=w321) -> ("Array u16"=w318:u16[], "Data Handle"=w323:u32, "error out"=w325:errorcluster)
                      n137 = Delete From Array(array=w318, length=2, index=0) -> (array with subset deleted=→"?":u16[])  [unwired: 1 out]
                    }
                  }
                }
                n138 = local write "Ready to Run"(FALSE ("PyLoN Ready")) -> ()
                n139 = call <userlib>:"ImageDestroy.vi"("error in"=w294, "Data handle"=w292) -> ()  [unwired: 1 out]
                n140 = stacked-sequence {
                  tunnel: w294 -> [w299]
                  tunnel: w293 -> [w298]
                  tunnel: [w297] -> w280
                  tunnel: [w296] -> w281
                  frame #0 {
                    n141 = call <userlib>:"CameraStop.vi"("error in"=w299, "Camera Handle"=w298) -> ("error out"=w297:errorcluster, "Camera Handle"=w296:u32)
                    n142 = call <vilib>:"Beep.vi"() -> ()  [unwired: 12 in]
                  }
                }
              }
            }
            "Ready to Run" <- TRUE
          }
          frame #1 {
            n143 = Equal?(x=w338, y=enum32{"RUN", "FOCUS", "FSRS", "SPECTROGRAPH"}."FOCUS") -> (x = y?=w334:bool)
            n144 = And(x=w334, y="?") -> (x .and. y?=w337:bool)
            n145 = case shown="True" w337 {
              tunnel: w330 -> [w346 w395]
              tunnel: [w342 w394] -> w333
              tunnel: w331 -> [w344 w393]
              tunnel: w336 -> [w345 w392]
              tunnel: [w343 w391] -> w332
              tunnel: w334 -> [w339 _]
              frame False {
                n146 = And(x=w339, y="?") -> (x .and. y?=w341:bool)
                n147 = case shown="False" w341 {
                  tunnel: w346 -> [w349 w375]
                  tunnel: w345 -> [w350 w374]
                  tunnel: w344 -> [w351 w373]
                  tunnel: [w347 w372] -> w343
                  tunnel: [w348 w371] -> w342
                  tunnel: w339 -> [w352 _]
                  frame False {
                    n148 = And(x=w352, y="?") -> (x .and. y?=w354:bool)
                    n149 = case shown="False" w354 {
                      tunnel: w351 -> [w355 w360]
                      tunnel: w350 -> [_ w363]
                      tunnel: w349 -> [w356 w362]
                      tunnel: [w356 w358] -> w348
                      tunnel: [w355 w359] -> w347
                      frame False {
                      }
                      frame True {
                        # "Acquire"
                        n150 = local read "FLIP SPECTRA"() -> (w365:bool)
                        n151 = Initialize Array(0.0, u32 1340) -> (w361:dbl[])
                        n152 = call "PyLoN_data.vi"("Number of Images"=w363, "error in (no error)"=w360, "PumpOffBkgd"=w361, "PumpOnBkgd"=w361, "Camera Handle"=w362) -> ("error out"=w359:errorcluster, "Camera Handle 2"=w358:u32, "Raman_Gain"=w357:dbl[])  [unwired: 1 in, 3 out]
                        n153 = case shown="False" w365 {
                          tunnel: w357 -> [w368 w370]
                          tunnel: [w368 w369] -> w364
                          frame False {
                          }
                          frame True {
                            n154 = Reciprocal(x=w370) -> (1/x=w369:dbl[])
                          }
                        }
                        n155 = local write "Spectra"(w364) -> ()
                      }
                    }
                  }
                  frame True {
                    # "Winspec"
                    n156 = while {
                      tunnel: w375 -> [w381]
                      tunnel: w374 -> [w382]
                      tunnel: [w376] -> w371
                      tunnel: w373 -> [w380]
                      tunnel: [w379] -> w372
                      stop <- w385 stop-if-true
                      n157 = local read item#11() -> (w385:bool)
                      n158 = Initialize Array(0.0, u32 1340) -> (w377:dbl[])
                      n159 = local read "FLIP SPECTRA"() -> (w384:bool)
                      n160 = call "PyLoN_data.vi"("Number of Images"=w382, "error in (no error)"=w380, "PumpOffBkgd"=w377, "PumpOnBkgd"=w377, "Camera Handle"=w381) -> ("error out"=w379:errorcluster, "Pump_Off"=w378:dbl[], "Camera Handle 2"=w376:u32)  [unwired: 1 in, 3 out]
                      n161 = case shown="False" w384 {
                        tunnel: w378 -> [w388 w389]
                        tunnel: [w388 w390] -> w383
                        frame False {
                        }
                        frame True {
                          n162 = Reciprocal(x=w389) -> (1/x=w390:dbl[])
                        }
                      }
                      n163 = local write "Spectra"(w383) -> ()
                    }
                  }
                }
              }
              frame True {
                # "Focus"
                n164 = while {
                  tunnel: w393 -> [w411]
                  tunnel: w392 -> [w412]
                  tunnel: [w410] -> w391
                  tunnel: w395 -> [w413]
                  tunnel: [w408] -> w394
                  stop <- "?" stop-if-true
                  n165 = property on="Spectra" class="WFGraph (strict)"("Active Cursor"=u32 1) -> (error out=w402:errorcluster)  [unwired: 2 in, 1 out]
                  n166 = property on="Spectra" class="WFGraph (strict)"("Active Cursor"=u32 0) -> (error out=w403:errorcluster)  [unwired: 2 in, 1 out]
                  n167 = Initialize Array(0.0, u32 1340) -> (w409:dbl[])
                  n168 = call "PyLoN_data.vi"("Number of Images"=w412, "error in (no error)"=w411, "PumpOffBkgd"=w409, "PumpOnBkgd"=w409, "Camera Handle"=w413) -> ("error out"=w410:errorcluster, "Camera Handle 2"=w408:u32, "Raman_Gain"=w407:dbl[], "x/y"=→"DATA LOOP":dbl)  [unwired: 1 in, 2 out]
                  n169 = property on="Spectra" class="WFGraph (strict)"(error in=w402) -> ("Cursor.Cursor Y"=w400:dbl)  [unwired: 1 in, 2 out]
                  n170 = property on="Spectra" class="WFGraph (strict)"(error in=w403) -> ("Cursor.Cursor Y"=w401:dbl)  [unwired: 1 in, 2 out]
                  n171 = local read "FLIP SPECTRA"() -> (w415:bool)
                  n172 = Subtract(x=w401, y=w400) -> (x-y=w399:dbl)
                  n173 = Absolute Value(x=w399) -> (abs(x)=w398:dbl)
                  n174 = Multiply(x=w398, y=100.0) -> (x*y=→"Gain":dbl)
                  n175 = case shown="False" w415 {
                    tunnel: w407 -> [w419 w421]
                    tunnel: [w419 w420] -> w414
                    frame False {
                    }
                    frame True {
                      n176 = Reciprocal(x=w421) -> (1/x=w420:dbl[])
                    }
                  }
                  "Spectra" <- w414
                }
              }
            }
          }
          frame #2 {
            n177 = Array Size(array=w424) -> (size(s)=w423:i32)
            n178 = Equal?(x=w434, y=enum32{"RUN", "FOCUS", "FSRS", "SPECTROGRAPH"}."FSRS") -> (x = y?=w432:bool)
            n179 = And(x="?", y=w432) -> (x .and. y?=w433:bool)
            n180 = case shown="False" w433 {
              tunnel: w431 -> [_ w444]
              tunnel: w428 -> [w435 w443]
              tunnel: w430 -> [w436 w439]
              tunnel: w424 -> [_ w442]
              tunnel: [w435 w441] -> w427
              tunnel: [w436 w440] -> w426
              tunnel: w425 -> [_ w438]
              tunnel: w423 -> [_ w437]
              frame False {
              }
              frame True {
                n181 = for {
                  N: w438 -> [_]
                  tunnel: w444 -> [w451]
                  tunnel: w443 -> [w450]
                  tunnel: w442 -> [w449]
                  tunnel: [w448] -> w441
                  tunnel: [w447] -> w440
                  tunnel: w439 -> [w446]
                  tunnel: w437 -> [w445]
                  n182 = stacked-sequence {
                    seq-local: [w454 _] -> [_ w464]
                    tunnel: w451 -> [_ w463]
                    tunnel: w450 -> [_ w462]
                    tunnel: [_ w458] -> _
                    tunnel: w449 -> [w452 w461]
                    tunnel: [_ w460] -> w447
                    tunnel: [_ w459] -> w448
                    tunnel: w446 -> [_ w458]
                    tunnel: w445 -> [_ w457]
                    frame #0 {
                      n183 = Array Size(array=w452) -> (size(s)=w456:i32)
                      n184 = call "randomize.vi"("Input array"=w452) -> ("Output array"=w453:dbl[])
                      n185 = Quotient & Remainder(x=w456, y="#Ground per set") -> (floor(x/y)=w454:u32)  [unwired: 1 out]
                      n186 = local write "Timepoints"(w453) -> ()
                    }
                    frame #1 {
                      n187 = for {
                        N: w457 -> [_]
                        tunnel: w464 -> [w471]
                        tunnel: w463 -> [w470]
                        tunnel: w462 -> [w469]
                        tunnel: w461 -> [w468]
                        tunnel: [w467] -> w460
                        tunnel: [w466] -> w459
                        tunnel: w458 -> [w465]
                        i -> [w472]
                        n188 = stacked-sequence {
                          seq-local: [w474 _] -> [_ w537]
                          seq-local: [w475 _] -> [_ w538]
                          seq-local: [w473 _] -> [_ w536]
                          tunnel: w472 -> [w476 w539]
                          tunnel: w471 -> [w481 _]
                          tunnel: w470 -> [w479 w541]
                          tunnel: w469 -> [w478 _]
                          tunnel: w465 -> [w477 _]
                          tunnel: w468 -> [_ w540]
                          tunnel: [_ w535] -> w467
                          tunnel: [_ w534] -> w466
                          frame #0 {
                            n189 = Quotient & Remainder(x=w476, y=w481) -> (x-y*floor(x/y)=w482:u32, floor(x/y)=w480:u32)
                            n190 = Equal To 0?(x=w482) -> (x = 0?=w483:bool)
                            n191 = case shown="True" w483 {
                              tunnel: w480 -> [_ w495]
                              tunnel: w479 -> [_ w499]
                              tunnel: w478 -> [w485 w498]
                              tunnel: w477 -> [w484 w497]
                              tunnel: [w485 w488] -> w474
                              tunnel: [w484 w487] -> w475
                              tunnel: w476 -> [_ w496]
                              tunnel: [_ w486] -> w473
                              frame False {
                              }
                              frame True {
                                n192 = flat-sequence {
                                tunnel: w499 -> [w520]
                                tunnel: w498 -> [w519]
                                tunnel: w497 -> [w518]
                                tunnel: w496 -> [w506]
                                tunnel: w495 -> [w504]
                                tunnel: [w517] -> w494
                                tunnel: [w516] -> w493
                                tunnel: [w513] -> w492
                                tunnel: [w512] -> w491
                                tunnel: [w501] -> w490
                                tunnel: [w500] -> w489
                                tunnel: w494 -> [w526]
                                tunnel: w493 -> [w525]
                                tunnel: w492 -> [w529]
                                tunnel: w491 -> [w528]
                                tunnel: w490 -> [w530]
                                tunnel: w489 -> [w524]
                                tunnel: [w526] -> w488
                                tunnel: [w525] -> w487
                                tunnel: [w524] -> w486
                                frame #0 {
                                w505 = "_" ("string")
                                n193 = local read "FLIP SPECTRA"() -> (w515:bool)
                                n194 = call "PyLoN_data.vi"("Number of Images"=w520, "error in (no error)"=w518, "Camera Handle"=w519) -> ("error out"=w516:errorcluster, "Pump_Off"=w512:dbl[], "Pump_On"=w513:dbl[], "Camera Handle 2"=w517:u32, "Raman_Gain"=w500:dbl[])  [unwired: 3 in, 1 out]
                                n195 = Format Into String(w506) -> (resulting string=w507:string)  [unwired: 3 in, 1 out]
                                n196 = Format Into String(w504) -> (resulting string=w503:string)  [unwired: 3 in, 1 out]
                                n197 = case shown="False" w515 {
                                tunnel: w500 -> [w521 w523]
                                tunnel: [w521 w522] -> w514
                                frame False {
                                }
                                frame True {
                                n198 = Reciprocal(x=w523) -> (1/x=w522:dbl[])
                                }
                                }
                                "?" <- w514
                                n199 = Path To String(path="File Path") -> (string=w511:string)
                                n200 = Concatenate Strings(w511, "\\" ("string"), "File Name", w505, w507, w505, w503, "gr" ("string")) -> (w501:string)
                                }
                                frame #1 {
                                n201 = String To Path(string=w530) -> (path=w531:path)
                                n202 = Build Array(w524, w529, w528) -> (w527:dbl[][])
                                n203 = call-poly <vilib>:"Write To Spreadsheet File.vi"("transpose? (no:F)"=TRUE, "format (%.3f)"="%.7f", "2D data"=w527, "file path (dialog if empty)"=w531) -> ()  [unwired: 4 in, 1 out]
                                }
                                }
                              }
                            }
                          }
                          frame #1 {
                            n204 = stacked-sequence {
                              seq-local: [_ w544 _ _ _] -> [_ _ _ w565 _]
                              seq-local: [_ w547 _ _ _] -> [_ _ _ w564 w571]
                              seq-local: [_ w546 _ _ _] -> [_ _ _ w563 _]
                              seq-local: [_ w545 _ _ _] -> [_ _ _ w562 _]
                              tunnel: w538 -> [_ w557 _ _ _]
                              tunnel: w537 -> [_ w556 _ _ _]
                              tunnel: w541 -> [_ w555 _ _ _]
                              tunnel: w540 -> [_ w552 _ _ _]
                              tunnel: w539 -> [_ w548 _ _ _]
                              tunnel: w536 -> [_ _ _ _ w572]
                              tunnel: [_ w543 _ _ _] -> w535
                              tunnel: [_ w542 _ _ _] -> w534
                              frame #0 {
                              }
                              frame #1 {
                                n205 = Index Array(array=w552, index=w548) -> (element=w551:dbl)
                                n206 = call "tppathcr.vi"("input"=w551) -> ("out"=w550:string)
                                n207 = local read "File Path"() -> (w554:path)
                                n208 = local read "File Name"() -> (w553:string)
                                n209 = call "PyLoN_data.vi"("Number of Images"=w555, "error in (no error)"=w557, "Camera Handle"=w556) -> ("error out"=w543:errorcluster, "Pump_Off"=w545:dbl[], "Pump_On"=w546:dbl[], "Camera Handle 2"=w542:u32, "Raman_Gain"=w547:dbl[])  [unwired: 3 in, 1 out]
                                n210 = Format Into String(w548) -> (resulting string=w558:string)  [unwired: 3 in, 1 out]
                                n211 = Path To String(path=w554) -> (string=w561:string)
                                n212 = Concatenate Strings(w561, "\\" ("string"), w553, "_" ("string"), w550, "exe" ("string"), w558) -> (w544:string)
                              }
                              frame #2 {
                              }
                              frame #3 {
                                n213 = String To Path(string=w565) -> (path=w567:path)
                                n214 = Build Array(w564, w563, w562) -> (w566:dbl[][])
                                n215 = call-poly <vilib>:"Write To Spreadsheet File.vi"("transpose? (no:F)"=TRUE, "format (%.3f)"="%.7f", "2D data"=w566, "file path (dialog if empty)"=w567) -> ()  [unwired: 4 in, 1 out]
                              }
                              frame #4 {
                                n216 = case shown="False" "Ground State\nSubstract?" {
                                tunnel: w572 -> [_ w581]
                                tunnel: w571 -> [w575 w580]
                                frame False {
                                n217 = local read "FLIP SPECTRA"() -> (w574:bool)
                                n218 = case shown="True" w574 {
                                tunnel: [w576 w578] -> w573
                                tunnel: w575 -> [w576 w577]
                                frame False {
                                }
                                frame True {
                                n219 = Reciprocal(x=w577) -> (1/x=w578:dbl[])
                                }
                                }
                                n220 = local write item#?(w573) -> ()
                                }
                                frame True {
                                n221 = local read "FLIP SPECTRA"() -> (w582:bool)
                                n222 = case shown="False" w582 {
                                tunnel: [w585 w590] -> w584
                                tunnel: w581 -> [w586 w587]
                                tunnel: [w586 w589] -> w583
                                tunnel: w580 -> [w585 w588]
                                frame False {
                                }
                                frame True {
                                n223 = Reciprocal(x=w588) -> (1/x=w590:dbl[])
                                n224 = Reciprocal(x=w587) -> (1/x=w589:dbl[])
                                }
                                }
                                n225 = Subtract(x=w584, y=w583) -> (x-y=w579:dbl[])
                                n226 = local write item#?(w579) -> ()
                                }
                                }
                              }
                            }
                          }
                        }
                      }
                    }
                  }
                }
              }
            }
          }
        }
        n227 = Or(x=w224, y="?") -> (x .or. y?=w226:bool)
      }
      n228 = property on="Run" class="TabCtl (strict)"("DisabledEnum"=T2."Enabled" ("Disabled")) -> ()  [unwired: 2 in, 2 out]
    }
    frame #2 {
      n229 = local read "Camera Handle"() -> (w591:u32)
      n230 = local read "error out"() -> (w592:errorcluster)
      n231 = local write "Ready to Run"(FALSE ("PyLoN Ready")) -> ()
      n232 = call "ExSubCloseCamUnInit.vi"("error in (no error)"=w592, "Camera Handle"=w591) -> ("error out"=w594:errorcluster)
      n233 = local write "error out"(w594) -> ()
    }
  }
